vi "Lab Panel V4.86.vi"() -> ()   [LabVIEW 2013] (continued)
                    n2581 = Unbundle(w4670) -> ("DESCRIPTION"=w4650:string)  [unwired: 4 out]
                    n2582 = Unbundle(w4669) -> ("DESCRIPTION"=w4649:string)  [unwired: 4 out]
                    n2583 = Unbundle(w4668) -> ("DESCRIPTION"=w4648:string)  [unwired: 4 out]
                    n2584 = Unbundle(w4665) -> ("DESCRIPTION"=w4645:string)  [unwired: 4 out]
                    n2585 = Unbundle(w4671) -> ("DESCRIPTION"=w4651:string)  [unwired: 4 out]
                    n2586 = Unbundle(w4667) -> ("DESCRIPTION"=w4647:string)  [unwired: 4 out]
                    n2587 = Unbundle(w4674) -> ("DESCRIPTION"=w4663:string)  [unwired: 4 out]
                    n2588 = Unbundle(w4672) -> ("DESCRIPTION"=w4652:string)  [unwired: 4 out]
                    n2589 = Unbundle(w4666) -> ("DESCRIPTION"=w4646:string)  [unwired: 4 out]
                    n2590 = Unbundle(w4673) -> ("DESCRIPTION"=w4653:string)  [unwired: 4 out]
                    n2591 = Concatenate Strings("[LAB05-2/", w4645) -> (w4635:string)
                    n2592 = Concatenate Strings("[LAB05-1/", w4646) -> (w4636:string)
                    n2593 = Concatenate Strings("[LAB04-2/", w4647) -> (w4637:string)
                    n2594 = Concatenate Strings("[LAB03-2/", w4649) -> (w4639:string)
                    n2595 = Concatenate Strings("[LAB04-1/", w4648) -> (w4638:string)
                    n2596 = Concatenate Strings("[LAB03-1/", w4650) -> (w4640:string)
                    n2597 = Concatenate Strings("[LAB01-2/", w4653) -> (w4643:string)
                    n2598 = Concatenate Strings("[LAB02-2/", w4651) -> (w4641:string)
                    n2599 = Concatenate Strings("[LAB01-1/", w4663) -> (w4644:string)
                    n2600 = Concatenate Strings("[LAB02-1/", w4652) -> (w4642:string)
                  }
                  frame #1 {
                    w4698 = "/"
                    w4699 = 2.0
                    n2601 = local read "DISP LAB01-2"() -> (w4778:T4)
                    n2602 = local read "DISP LAB01-1"() -> (w4779:T4)
                    n2603 = local read "DISP LAB02-1"() -> (w4777:T4)
                    n2604 = local read "DISP LAB03-2"() -> (w4774:T4)
                    n2605 = local read "DISP LAB02-2"() -> (w4776:T4)
                    n2606 = local read "DISP LAB03-1"() -> (w4775:T4)
                    n2607 = local read "DISP LAB04-2"() -> (w4772:T4)
                    n2608 = local read "DISP LAB04-1"() -> (w4773:T4)
                    n2609 = local read "DISP LAB05-1"() -> (w4771:T4)
                    n2610 = local read "DISP LAB05-2"() -> (w4770:T4)
                    n2611 = Unbundle(w4778) -> ("CYCLE"=w4762:dbl, "MINS"=w4761:dbl, "STATUS"=w4758:string)
                    n2612 = Unbundle(w4779) -> ("CYCLE"=w4767:dbl, "MINS"=w4766:dbl, "STATUS"=w4763:string)
                    n2613 = Unbundle(w4777) -> ("CYCLE"=w4755:dbl, "MINS"=w4754:dbl, "STATUS"=w4753:string)
                    n2614 = Unbundle(w4774) -> ("CYCLE"=w4742:dbl, "MINS"=w4741:dbl, "STATUS"=w4738:string)
                    n2615 = Unbundle(w4775) -> ("CYCLE"=w4747:dbl, "MINS"=w4746:dbl, "STATUS"=w4743:string)
                    n2616 = Unbundle(w4776) -> ("CYCLE"=w4752:dbl, "MINS"=w4751:dbl, "STATUS"=w4748:string)
                    n2617 = Unbundle(w4773) -> ("CYCLE"=w4737:dbl, "MINS"=w4736:dbl, "STATUS"=w4733:string)
                    n2618 = Unbundle(w4772) -> ("CYCLE"=w4732:dbl, "MINS"=w4731:dbl, "STATUS"=w4728:string)
                    n2619 = Unbundle(w4771) -> ("CYCLE"=w4727:dbl, "MINS"=w4726:dbl, "STATUS"=w4723:string)
                    n2620 = Unbundle(w4770) -> ("CYCLE"=w4769:dbl, "MINS"=w4768:dbl, "STATUS"=w4720:string)
                    n2621 = Number To Decimal String(number=w4755) -> (decimal integer string=w4757:string)  [unwired: 1 in]
                    n2622 = Number To Decimal String(number=w4752) -> (decimal integer string=w4750:string)  [unwired: 1 in]
                    n2623 = Number To Decimal String(number=w4747) -> (decimal integer string=w4745:string)  [unwired: 1 in]
                    n2624 = Number To Decimal String(number=w4762) -> (decimal integer string=w4760:string)  [unwired: 1 in]
                    n2625 = Number To Decimal String(number=w4742) -> (decimal integer string=w4740:string)  [unwired: 1 in]
                    n2626 = Number To Decimal String(number=w4767) -> (decimal integer string=w4765:string)  [unwired: 1 in]
                    n2627 = Number To Decimal String(number=w4769) -> (decimal integer string=w4722:string)  [unwired: 1 in]
                    n2628 = Number To Decimal String(number=w4737) -> (decimal integer string=w4735:string)  [unwired: 1 in]
                    n2629 = Number To Decimal String(number=w4732) -> (decimal integer string=w4730:string)  [unwired: 1 in]
                    n2630 = Number To Decimal String(number=w4727) -> (decimal integer string=w4725:string)  [unwired: 1 in]
                    n2631 = Number To Fractional String(number=w4754, precision (6)=w4699) -> (F-format string=w4756:string)  [unwired: 2 in]
                    n2632 = Number To Fractional String(number=w4741, precision (6)=w4699) -> (F-format string=w4739:string)  [unwired: 2 in]
                    n2633 = Number To Fractional String(number=w4751, precision (6)=w4699) -> (F-format string=w4749:string)  [unwired: 2 in]
                    n2634 = Number To Fractional String(number=w4746, precision (6)=w4699) -> (F-format string=w4744:string)  [unwired: 2 in]
                    n2635 = Number To Fractional String(number=w4731, precision (6)=w4699) -> (F-format string=w4729:string)  [unwired: 2 in]
                    n2636 = Number To Fractional String(number=w4736, precision (6)=w4699) -> (F-format string=w4734:string)  [unwired: 2 in]
                    n2637 = Number To Fractional String(number=w4761, precision (6)=w4699) -> (F-format string=w4759:string)  [unwired: 2 in]
                    n2638 = Number To Fractional String(number=w4726, precision (6)=w4699) -> (F-format string=w4724:string)  [unwired: 2 in]
                    n2639 = Number To Fractional String(number=w4766, precision (6)=w4699) -> (F-format string=w4764:string)  [unwired: 2 in]
                    n2640 = Number To Fractional String(number=w4768, precision (6)=w4699) -> (F-format string=w4721:string)  [unwired: 2 in]
                    n2641 = Concatenate Strings(w4698, w4740, w4698, w4739, w4698, w4738) -> (w4714:string)
                    n2642 = Concatenate Strings(w4698, w4735, w4698, w4734, w4698, w4733) -> (w4713:string)
                    n2643 = Concatenate Strings(w4698, w4730, w4698, w4729, w4698, w4728) -> (w4712:string)
                    n2644 = Concatenate Strings(w4698, w4725, w4698, w4724, w4698, w4723) -> (w4711:string)
                    n2645 = Concatenate Strings(w4698, w4722, w4698, w4721, w4698, w4720) -> (w4710:string)
                    n2646 = Concatenate Strings(w4698, w4765, w4698, w4764, w4698, w4763) -> (w4719:string)
                    n2647 = Concatenate Strings(w4698, w4745, w4698, w4744, w4698, w4743) -> (w4715:string)
                    n2648 = Concatenate Strings(w4698, w4760, w4698, w4759, w4698, w4758) -> (w4718:string)
                    n2649 = Concatenate Strings(w4698, w4757, w4698, w4756, w4698, w4753) -> (w4717:string)
                    n2650 = Concatenate Strings(w4698, w4750, w4698, w4749, w4698, w4748) -> (w4716:string)
                    n2651 = Concatenate Strings("]", "\r") -> (w4695:string)
                    n2652 = Concatenate Strings(w4690, w4715, w4695) -> (w4705:string)
                    n2653 = Concatenate Strings(w4692, w4717, w4695) -> (w4707:string)
                    n2654 = Concatenate Strings(w4691, w4716, w4695) -> (w4706:string)
                    n2655 = Concatenate Strings(w4687, w4712, w4695) -> (w4702:string)
                    n2656 = Concatenate Strings(w4688, w4711, w4695) -> (w4703:string)
                    n2657 = Concatenate Strings(w4686, w4713, w4695) -> (w4701:string)
                    n2658 = Concatenate Strings(w4685, w4714, w4695) -> (w4700:string)
                    n2659 = Concatenate Strings(w4689, w4710, w4695) -> (w4704:string)
                    n2660 = Concatenate Strings(w4693, w4718, w4695) -> (w4708:string)
                    n2661 = Concatenate Strings(w4694, w4719, w4695) -> (w4709:string)
                    n2662 = Concatenate Strings(w4709, w4708, w4707, w4706, w4705, w4700, w4701, w4702, w4703, w4704) -> (w4678:string)
                    n2663 = Concatenate Strings("[PANEL/", "DESC/", "CYCLES/", "MINS/", "STATUS]", "\r", w4678) -> (w4677:string)
                    "MAIL REPORT" <- w4677
                    n2664 = global write "Global display 3.vi" "log all"(w4677) -> ()
                  }
                  frame #2 {
                    w4808 = "END"
                    n2665 = local read "mail control"() -> (w4809:string)
                    n2666 = case shown="False" w4804 {
                      tunnel: w4809 -> [w4833 _]
                      tunnel: w4808 -> [w4832 _]
                      tunnel: [w4831 FALSE] -> w4794
                      frame False {
                        n2667 = Equal?(x=w4833, y=w4832) -> (x = y?=w4831:bool)
                      }
                      frame True {
                      }
                    }
                    n2668 = case shown="False" w4810 {
                      tunnel: w4809 -> [w4849 _]
                      tunnel: w4808 -> [w4848 _]
                      tunnel: [w4847 FALSE] -> w4798
                      frame False {
                        n2669 = Equal?(x=w4849, y=w4848) -> (x = y?=w4847:bool)
                      }
                      frame True {
                      }
                    }
                    n2670 = case shown="False" w4807 {
                      tunnel: w4809 -> [w4845 _]
                      tunnel: w4808 -> [w4844 _]
                      tunnel: [w4843 FALSE] -> w4797
                      frame False {
                        n2671 = Equal?(x=w4845, y=w4844) -> (x = y?=w4843:bool)
                      }
                      frame True {
                      }
                    }
                    n2672 = case shown="False" w4805 {
                      tunnel: w4809 -> [w4837 _]
                      tunnel: w4808 -> [w4836 _]
                      tunnel: [w4835 FALSE] -> w4795
                      frame False {
                        n2673 = Equal?(x=w4837, y=w4836) -> (x = y?=w4835:bool)
                      }
                      frame True {
                      }
                    }
                    n2674 = case shown="False" w4806 {
                      tunnel: w4809 -> [w4841 _]
                      tunnel: w4808 -> [w4840 _]
                      tunnel: [w4839 FALSE] -> w4796
                      frame False {
                        n2675 = Equal?(x=w4841, y=w4840) -> (x = y?=w4839:bool)
                      }
                      frame True {
                      }
                    }
                    n2676 = Or(x=w4796, y=w4795) -> (x .or. y?=w4787:bool)
                    n2677 = Or(x=w4798, y=w4797) -> (x .or. y?=w4788:bool)
                    n2678 = Or(x=w4788, y=w4787) -> (x .or. y?=w4783:bool)
                    n2679 = case shown="False" w4800 {
                      tunnel: w4809 -> [w4817 _]
                      tunnel: w4808 -> [w4816 _]
                      tunnel: [w4815 FALSE] -> w4789
                      frame False {
                        n2680 = Equal?(x=w4817, y=w4816) -> (x = y?=w4815:bool)
                      }
                      frame True {
                      }
                    }
                    n2681 = case shown="False" w4799 {
                      tunnel: w4809 -> [w4813 _]
                      tunnel: w4808 -> [w4812 _]
                      tunnel: [w4811 FALSE] -> w4793
                      frame False {
                        n2682 = Equal?(x=w4813, y=w4812) -> (x = y?=w4811:bool)
                      }
                      frame True {
                      }
                    }
                    n2683 = case shown="False" w4801 {
                      tunnel: w4809 -> [w4821 _]
                      tunnel: w4808 -> [w4820 _]
                      tunnel: [w4819 FALSE] -> w4790
                      frame False {
                        n2684 = Equal?(x=w4821, y=w4820) -> (x = y?=w4819:bool)
                      }
                      frame True {
                      }
                    }
                    n2685 = case shown="False" w4803 {
                      tunnel: w4809 -> [w4829 _]
                      tunnel: w4808 -> [w4828 _]
                      tunnel: [w4827 FALSE] -> w4792
                      frame False {
                        n2686 = Equal?(x=w4829, y=w4828) -> (x = y?=w4827:bool)
                      }
                      frame True {
                      }
                    }
                    n2687 = case shown="False" w4802 {
                      tunnel: w4809 -> [w4825 _]
                      tunnel: w4808 -> [w4824 _]
                      tunnel: [w4823 FALSE] -> w4791
                      frame False {
                        n2688 = Equal?(x=w4825, y=w4824) -> (x = y?=w4823:bool)
                      }
                      frame True {
                      }
                    }
                    n2689 = Or(x=w4792, y=w4791) -> (x .or. y?=w4786:bool)
                    n2690 = Or(x=w4790, y=w4789) -> (x .or. y?=w4785:bool)
                    n2691 = Or(x=w4793, y=w4794) -> (x .or. y?=w4781:bool)
                    n2692 = Or(x=w4786, y=w4785) -> (x .or. y?=w4784:bool)
                    n2693 = Or(x=w4783, y=w4784) -> (x .or. y?=w4782:bool)
                    n2694 = Or(x=w4782, y=w4781) -> (x .or. y?=w4780:bool)
                  }
                  frame #3 {
                    n2695 = local read "on loops"() -> (w4863:dbl)
                    n2696 = local read "jig cycle"() -> (w4860:dbl)
                    n2697 = local read "Send Mail Now"() -> (w4854:bool)
                    n2698 = Add(x=w4863, y=3.0) -> (x+y=w4861:dbl)
                    n2699 = Equal?(x=w4860, y=w4861) -> (x = y?=w4855:bool)
                    n2700 = And(x=w4855, y=w4854) -> (x .and. y?=w4853:bool)
                    n2701 = And(x=w4859, y=w4855) -> (x .and. y?=w4858:bool)
                    n2702 = And(x=w4858, y=w4857) -> (x .and. y?=w4856:bool)
                    n2703 = Or(x=w4856, y=w4853) -> (x .or. y?=w4852:bool)
                    n2704 = case shown="True" w4852 {
                      tunnel: w4868 -> [_ w4874]
                      tunnel: w4867 -> [_ w4873]
                      tunnel: "Lab Panel Test Status" -> [_ w4872]
                      tunnel: w4865 -> [_ w4871]
                      tunnel: w4864 -> [_ w4870]
                      tunnel: w4851 -> [_ w4869]
                      frame False {
                      }
                      frame True {
                        n2705 = stacked-sequence {
                          tunnel: w4874 -> [w4882 _]
                          tunnel: w4873 -> [w4881 _]
                          tunnel: w4872 -> [w4880 _]
                          tunnel: w4871 -> [w4879 _]
                          tunnel: w4870 -> [w4878 _]
                          tunnel: w4869 -> [w4877 _]
                          frame #0 {
                            n2706 = call "sub vi - send mail v5.vi"("TO:"=w4882, "subject"=w4880, "from"=w4878, "out going server"=w4879, "message"=w4881) -> ("error out"=w4876:errorcluster)  [unwired: 10 in]
                            n2707 = Bundle(cluster=w4877, "mail error"=w4876) -> (w4875:T6)  [unwired: 6 in]
                            n2708 = local write "MAIL SETTINGS"(w4875) -> ()
                          }
                          frame #1 {
                            n2709 = local write "mail control"("") -> ()
                            n2710 = local write "Send Mail Now"(FALSE) -> ()
                          }
                        }
                      }
                    }
                  }
                }
              }
            }
          }
          frame #18 {
            # "save jig cycle values once all run switches are off"
            n2711 = stacked-sequence {
              tunnel: w4894 -> [_ w4923]
              tunnel: w4893 -> [_ w4922]
              tunnel: w4892 -> [_ w4921]
              tunnel: w4891 -> [_ w4920]
              tunnel: w4890 -> [_ w4919]
              tunnel: w4889 -> [_ w4918]
              tunnel: w4888 -> [_ w4917]
              tunnel: w4887 -> [_ w4916]
              tunnel: w4886 -> [_ w4915]
              tunnel: w4885 -> [_ w4914]
              frame #0 {
              }
              frame #1 {
                n2712 = Not(x=w4914) -> (.not. x?=w4897:bool)
                n2713 = Not(x=w4922) -> (.not. x?=w4912:bool)
                n2714 = Not(x=w4919) -> (.not. x?=w4907:bool)
                n2715 = Not(x=w4917) -> (.not. x?=w4903:bool)
                n2716 = Not(x=w4915) -> (.not. x?=w4899:bool)
                n2717 = Not(x=w4923) -> (.not. x?=w4913:bool)
                n2718 = Not(x=w4921) -> (.not. x?=w4911:bool)
                n2719 = Not(x=w4918) -> (.not. x?=w4905:bool)
                n2720 = Not(x=w4920) -> (.not. x?=w4909:bool)
                n2721 = Not(x=w4916) -> (.not. x?=w4901:bool)
                n2722 = local read "Save JC"() -> (w4925:bool)
                n2723 = And(x=w4913, y=w4912) -> (x .and. y?=w4910:bool)
                n2724 = And(x=w4910, y=w4911) -> (x .and. y?=w4908:bool)
                n2725 = And(x=w4908, y=w4909) -> (x .and. y?=w4906:bool)
                n2726 = And(x=w4906, y=w4907) -> (x .and. y?=w4904:bool)
                n2727 = And(x=w4904, y=w4905) -> (x .and. y?=w4902:bool)
                n2728 = And(x=w4902, y=w4903) -> (x .and. y?=w4900:bool)
                n2729 = And(x=w4900, y=w4901) -> (x .and. y?=w4898:bool)
                n2730 = And(x=w4898, y=w4899) -> (x .and. y?=w4896:bool)
                n2731 = And(x=w4896, y=w4897) -> (x .and. y?=w4895:bool)
                n2732 = And(x=w4895, y=w4925) -> (x .and. y?=w4924:bool)
                n2733 = case shown="True" w4924 {
                  tunnel: w4895 -> [w4926 _]
                  frame False {
                    n2734 = case shown="False" w4926 {
                      frame False {
                        n2735 = local write "Save JC"(TRUE) -> ()
                      }
                      frame True {
                      }
                    }
                  }
                  frame True {
                    n2736 = stacked-sequence {
                      frame #0 {
                        n2737 = String To Path(string="c:\\crabtree\\Jig Cycles\\") -> (path=w4938:path)
                        n2738 = Build Path(base path=w4938, name or relative path="jigcycles.bin") -> (appended path=w4936:path)
                        n2739 = Create Folder(path (use dialog)=w4938) -> (error out=w4940:errorcluster)  [unwired: 2 in, 2 out]
                        n2740 = local read "JIG RELAY CYCLES"() -> (w4930:T7)
                        n2741 = call <vilib>:"Clear Errors.vi"("error in (no error)"=w4940) -> ()  [unwired: 6 in, 1 out]
                        n2742 = local write "Save JC"(FALSE) -> ()
                        n2743 = Open/Create/Replace File(file path (use dialog)=w4936, operation (0:open)=T19."replace or create") -> (refnum out=w4934:refnum<file>, error out=w4935:errorcluster)  [unwired: 4 in, 1 out]
                        n2744 = Write to Binary File(file (use dialog)=w4934, data=w4930, error in=w4935) -> (refnum out=w4933:refnum<file>, error out=w4932:errorcluster)  [unwired: 3 in, 1 out]
                        n2745 = Close File(refnum=w4933, error in=w4932) -> (error out=w4931:errorcluster)  [unwired: 1 out]
                        n2746 = local write "data file error"(w4931) -> ()
                      }
                      frame #1 {
                        n2747 = local read "JIG RELAY CYCLES"() -> (w4963:T7)
                        n2748 = Unbundle By Name(w4963) -> ("LAB01-1"=w4958:dbl, "LAB01-2"=w4957:dbl, "LAB02-1"=w4955:dbl, "LAB02-2"=w4954:dbl, "LAB03-1"=w4952:dbl, "LAB03-2"=w4949:dbl, "LAB04-1"=w4948:dbl, "LAB04-2"=w4946:dbl, "LAB05-1"=w4944:dbl, "LAB05-2"=w4942:dbl)
                        n2749 = stacked-sequence {
                          tunnel: w4958 -> [w4966 _ _ _ _ _ _ _ _ _]
                          tunnel: 1000000 -> [w4969 w4979 w4989 w4999 w5009 w5019 w5029 w5039 w5049 w5059]
                          tunnel: [w4967 _ _ _ _ _ _ _ _ _] -> w4961
                          tunnel: "TEST STATION HAS REACHED 1 MILLION CYCLES, REPLACE  CONTROL RELAYS" -> [w4965 w4977 w4987 w4997 w5007 w5017 w5027 w5037 w5047 w5057]
                          tunnel: [_ w4976 _ _ _ _ _ _ _ _] -> w4959
                          tunnel: w4957 -> [_ w4975 _ _ _ _ _ _ _ _]
                          tunnel: [_ _ w4986 _ _ _ _ _ _ _] -> w4956
                          tunnel: w4955 -> [_ _ w4985 _ _ _ _ _ _ _]
                          tunnel: w4954 -> [_ _ _ w4996 _ _ _ _ _ _]
                          tunnel: [_ _ _ w4995 _ _ _ _ _ _] -> w4953
                          tunnel: w4952 -> [_ _ _ _ w5006 _ _ _ _ _]
                          tunnel: [_ _ _ _ w5005 _ _ _ _ _] -> w4951
                          tunnel: [_ _ _ _ _ w5016 _ _ _ _] -> w4950
                          tunnel: w4949 -> [_ _ _ _ _ w5015 _ _ _ _]
                          tunnel: w4948 -> [_ _ _ _ _ _ w5026 _ _ _]
                          tunnel: [_ _ _ _ _ _ w5025 _ _ _] -> w4947
                          tunnel: w4946 -> [_ _ _ _ _ _ _ w5036 _ _]
                          tunnel: [_ _ _ _ _ _ _ w5035 _ _] -> w4945
                          tunnel: w4944 -> [_ _ _ _ _ _ _ _ w5046 _]
                          tunnel: [_ _ _ _ _ _ _ _ w5045 _] -> w4943
                          tunnel: w4942 -> [_ _ _ _ _ _ _ _ _ w5056]
                          tunnel: [_ _ _ _ _ _ _ _ _ w5055] -> w4941
                          frame #0 {
                            n2750 = Greater?(x=w4966, y=w4969) -> (0:w4968:bool)
                            n2751 = case shown="True" w4968 {
                              tunnel: [w4970 0] -> w4967
                              tunnel: w4966 -> [w4970 _]
                              tunnel: w4965 -> [_ w4971]
                              frame False {
                              }
                              frame True {
                                n2752 = Concatenate Strings("LA01-1 ", w4971) -> (w4974:string)
                                n2753 = One Button Dialog(message=w4974) -> ()  [unwired: 1 in, 1 out]
                              }
                            }
                          }
                          frame #1 {
                            n2754 = Greater?(x=w4975, y=w4979) -> (0:w4978:bool)
                            n2755 = case shown="True" w4978 {
                              tunnel: [w4980 0] -> w4976
                              tunnel: w4975 -> [w4980 _]
                              tunnel: w4977 -> [_ w4981]
                              frame False {
                              }
                              frame True {
                                n2756 = Concatenate Strings("LA01-2 ", w4981) -> (w4984:string)
                                n2757 = One Button Dialog(message=w4984) -> ()  [unwired: 1 in, 1 out]
                              }
                            }
                          }
                          frame #2 {
                            n2758 = Greater?(x=w4985, y=w4989) -> (0:w4988:bool)
                            n2759 = case shown="True" w4988 {
                              tunnel: [w4990 0] -> w4986
                              tunnel: w4985 -> [w4990 _]
                              tunnel: w4987 -> [_ w4991]
                              frame False {
                              }
                              frame True {
                                n2760 = Concatenate Strings("LA02-1 ", w4991) -> (w4994:string)
                                n2761 = One Button Dialog(message=w4994) -> ()  [unwired: 1 in, 1 out]
                              }
                            }
                          }
                          frame #3 {
                            n2762 = Greater?(x=w4996, y=w4999) -> (0:w4998:bool)
                            n2763 = case shown="True" w4998 {
                              tunnel: [w5000 0] -> w4995
                              tunnel: w4996 -> [w5000 _]
                              tunnel: w4997 -> [_ w5001]
                              frame False {
                              }
                              frame True {
                                n2764 = Concatenate Strings("LA02-2 ", w5001) -> (w5004:string)
                                n2765 = One Button Dialog(message=w5004) -> ()  [unwired: 1 in, 1 out]
                              }
                            }
                          }
                          frame #4 {
                            n2766 = Greater?(x=w5006, y=w5009) -> (0:w5008:bool)
                            n2767 = case shown="True" w5008 {
                              tunnel: [w5010 0] -> w5005
                              tunnel: w5006 -> [w5010 _]
                              tunnel: w5007 -> [_ w5011]
                              frame False {
                              }
                              frame True {
                                n2768 = Concatenate Strings("LA03-1 ", w5011) -> (w5014:string)
                                n2769 = One Button Dialog(message=w5014) -> ()  [unwired: 1 in, 1 out]
                              }
                            }
                          }
                          frame #5 {
                            n2770 = Greater?(x=w5015, y=w5019) -> (0:w5018:bool)
                            n2771 = case shown="True" w5018 {
                              tunnel: [w5020 0] -> w5016
                              tunnel: w5015 -> [w5020 _]
                              tunnel: w5017 -> [_ w5021]
                              frame False {
                              }
                              frame True {
                                n2772 = Concatenate Strings("LA03-2 ", w5021) -> (w5024:string)
                                n2773 = One Button Dialog(message=w5024) -> ()  [unwired: 1 in, 1 out]
                              }
                            }
                          }
                          frame #6 {
                            n2774 = Greater?(x=w5026, y=w5029) -> (0:w5028:bool)
                            n2775 = case shown="True" w5028 {
                              tunnel: [w5030 0] -> w5025
                              tunnel: w5026 -> [w5030 _]
                              tunnel: w5027 -> [_ w5031]
                              frame False {
                              }
                              frame True {
                                n2776 = Concatenate Strings("LA04-1 ", w5031) -> (w5034:string)
                                n2777 = One Button Dialog(message=w5034) -> ()  [unwired: 1 in, 1 out]
                              }
                            }
                          }
                          frame #7 {
                            n2778 = Greater?(x=w5036, y=w5039) -> (0:w5038:bool)
                            n2779 = case shown="True" w5038 {
                              tunnel: [w5040 0] -> w5035
                              tunnel: w5036 -> [w5040 _]
                              tunnel: w5037 -> [_ w5041]
                              frame False {
                              }
                              frame True {
                                n2780 = Concatenate Strings("LA04-2 ", w5041) -> (w5044:string)
                                n2781 = One Button Dialog(message=w5044) -> ()  [unwired: 1 in, 1 out]
                              }
                            }
                          }
                          frame #8 {
                            n2782 = Greater?(x=w5046, y=w5049) -> (0:w5048:bool)
                            n2783 = case shown="True" w5048 {
                              tunnel: [w5050 0] -> w5045
                              tunnel: w5046 -> [w5050 _]
                              tunnel: w5047 -> [_ w5051]
                              frame False {
                              }
                              frame True {
                                n2784 = Concatenate Strings("LA05-1 ", w5051) -> (w5054:string)
                                n2785 = One Button Dialog(message=w5054) -> ()  [unwired: 1 in, 1 out]
                              }
                            }
                          }
                          frame #9 {
                            n2786 = Greater?(x=w5056, y=w5059) -> (0:w5058:bool)
                            n2787 = case shown="True" w5058 {
                              tunnel: [w5060 0] -> w5055
                              tunnel: w5056 -> [w5060 _]
                              tunnel: w5057 -> [_ w5061]
                              frame False {
                              }
                              frame True {
                                n2788 = Concatenate Strings("LA05-2 ", w5061) -> (w5064:string)
                                n2789 = One Button Dialog(message=w5064) -> ()  [unwired: 1 in, 1 out]
                              }
                            }
                          }
                        }
                        n2790 = Bundle By Name(cluster=w4963, "LAB01-1"=w4961, "LAB01-2"=w4959, "LAB02-1"=w4956, "LAB02-2"=w4953, "LAB03-1"=w4951, "LAB03-2"=w4950, "LAB04-1"=w4947, "LAB04-2"=w4945, "LAB05-1"=w4943, "LAB05-2"=w4941) -> (w4962:T7)
                        n2791 = local write "JIG RELAY CYCLES"(w4962) -> ()
                      }
                    }
                  }
                }
              }
            }
          }
          frame #19 {
            # "get temperature values"
            n2792 = local read "simulate"() -> (w5077:bool)
            n2793 = local read "Temp Test Cal"() -> (w5074:dbl)
            n2794 = stacked-sequence {
              tunnel: w5077 -> [_ w5133 w5178 w5223 w5268 w5313]
              tunnel: T12 {"1  (A) cal"=1.0, "1 (V) cal"=1.0, "1 (PF) cal"=1.0, "1 (TL) cal"=1.0, "1 (TN) cal"=1.0, "2 (A) cal"=1.0, "2 (V) cal"=1.0, "2 (PF) cal"=1.0, "2 (TL) cal"=1.0, "2 (TN) cal"=1.0} ("CAL LAB01") -> [_ w5132 w5177 w5222 w5267 w5312]
              tunnel: w5075 -> [_ w5130 _ _ _ _]
              tunnel: w5074 -> [_ w5126 w5176 w5221 w5266 w5311]
              tunnel: w5073 -> [_ w5121 _ _ _ _]
              tunnel: w5072 -> [_ _ w5167 _ _ _]
              tunnel: w5071 -> [_ _ w5166 _ _ _]
              tunnel: w5070 -> [_ _ _ w5212 _ _]
              tunnel: w5069 -> [_ _ _ w5211 _ _]
              tunnel: w5068 -> [_ _ _ _ w5257 _]
              tunnel: w5067 -> [_ _ _ _ w5256 _]
              tunnel: w5066 -> [_ _ _ _ _ w5302]
              tunnel: w5065 -> [_ _ _ _ _ w5301]
              frame #0 {
                n2795 = local read "Select COM port"() -> (w5082:refnum<visa-resource-name>)
                "COM port" <- w5082
                n2796 = local read "jig cycle"() -> (w5083:dbl)
                n2797 = local read "on loops"() -> (w5085:dbl)
                n2798 = global write "Global 1.vi" "tmp dly lps"("Temp Delay Lps") -> ()
                n2799 = global write "Global 1.vi" "dly value"("Temp Value") -> ()
                n2800 = Add(x=w5085, y=3) -> (x+y=w5086:dbl)
                n2801 = global write "Global 1.vi" "COM port"(w5082) -> ()
                n2802 = Equal?(x=w5083, y=w5086) -> (x = y?=w5079:bool)
                n2803 = local read "Temp Loops"() -> (w5078:dbl)
                n2804 = case shown="True" w5079 {
                  tunnel: w5078 -> [_ w5088]
                  frame False {
                  }
                  frame True {
                    n2805 = stacked-sequence {
                      tunnel: w5088 -> [w5091 w5119]
                      frame #0 {
                        n2806 = local read "simulate"() -> (w5089:bool)
                        n2807 = case shown="5" w5091 {
                          tunnel: 1.0 -> [_ w5096 w5098 w5104 w5108 w5113]
                          tunnel: w5089 -> [_ w5092 w5097 w5102 w5109 w5112]
                          frame 0, Default {
                          }
                          frame 1 {
                            w5094 = FALSE
                            n2808 = call "sub vi - GET ALL TEMP v5.vi"("LA01-EN"=TRUE, "simulate"=w5092, "LA02-EN"=w5094, "LA03-EN"=w5094, "LA04-EN"=w5094, "LA05-EN"=w5094, "Gen Cal Value"=w5096) -> ("LA01 TEMP"=w5093:T22)  [unwired: 3 in, 5 out]
                            n2809 = local write "LAB01 TEMP"(w5093) -> ()
                          }
                          frame 2 {
                            w5099 = FALSE
                            n2810 = call "sub vi - GET ALL TEMP v5.vi"("LA01-EN"=w5099, "simulate"=w5097, "LA02-EN"=TRUE, "LA03-EN"=w5099, "LA04-EN"=w5099, "LA05-EN"=w5099, "Gen Cal Value"=w5098) -> ("LA02 TEMP"=w5101:T22)  [unwired: 3 in, 5 out]
                            n2811 = local write "LAB02 TEMP"(w5101) -> ()
                          }
                          frame 3 {
                            w5105 = FALSE
                            n2812 = call "sub vi - GET ALL TEMP v5.vi"("LA01-EN"=w5105, "simulate"=w5102, "LA02-EN"=w5105, "LA03-EN"=TRUE, "LA04-EN"=w5105, "LA05-EN"=w5105, "Gen Cal Value"=w5104) -> ("LA03 TEMP"=w5103:T22)  [unwired: 3 in, 5 out]
                            n2813 = local write "LAB03 TEMP"(w5103) -> ()
                          }
                          frame 4 {
                            w5110 = FALSE
                            n2814 = call "sub vi - GET ALL TEMP v5.vi"("LA01-EN"=w5110, "simulate"=w5109, "LA02-EN"=w5110, "LA03-EN"=w5110, "LA04-EN"=TRUE, "LA05-EN"=w5110, "Gen Cal Value"=w5108) -> ("LA04 TEMP"=w5107:T22)  [unwired: 3 in, 5 out]
                            n2815 = local write "LAB04 TEMP"(w5107) -> ()
                          }
                          frame 5 {
                            w5115 = FALSE
                            n2816 = call "sub vi - GET ALL TEMP v5.vi"("LA01-EN"=w5115, "simulate"=w5112, "LA02-EN"=w5115, "LA03-EN"=w5115, "LA04-EN"=w5115, "LA05-EN"=TRUE, "Gen Cal Value"=w5113) -> ("LA05 TEMP"=w5114:T22)  [unwired: 3 in, 5 out]
                            n2817 = local write "LAB05 TEMP"(w5114) -> ()
                          }
                        }
                      }
                      frame #1 {
                        n2818 = Greater Or Equal?(x=w5119, y=5) -> (x >= y?=w5117:bool)
                        n2819 = case shown="True" w5117 {
                          frame False {
                          }
                          frame True {
                            n2820 = local write "Temp Loops"(0) -> ()
                          }
                        }
                      }
                    }
                    n2821 = local write "TEMP"(TRUE) -> ()
                  }
                }
              }
              frame #1 {
                n2822 = case shown="False" w5133 {
                  tunnel: [w5164 w5165] -> w5149
                  tunnel: w5132 -> [_ w5165]
                  frame False {
                    n2823 = local read "CAL LAB01"() -> (w5164:T12)
                  }
                  frame True {
                  }
                }
                n2824 = local read "LAB01 TEMP"() -> (w5139:T11)
                n2825 = local read "TEMP LA01"() -> (w5140:T8)
                n2826 = call "sub vi - temperature delay v2.vi"("temp values IN"=w5140, "temp signals"=w5139) -> ("T2-N"=w5135:dbl, "T2-L"=w5136:dbl, "T1-N"=w5137:dbl, "T1-L"=w5138:dbl, "temp values OUT"=w5134:T40)  [unwired: 5 in]
                n2827 = Unbundle By Name(w5149) -> ("1 (TL) cal"=w5144:dbl, "1 (TN) cal"=w5143:dbl, "2 (TL) cal"=w5142:dbl, "2 (TN) cal"=w5141:dbl)  [unwired: 6 out]
                n2828 = local write "TEMP LA01"(w5134) -> ()
                n2829 = Multiply(x=w5138, y=w5144) -> (x*y=w5131:dbl)
                n2830 = Multiply(x=w5137, y=w5143) -> (x*y=w5128:dbl)
                n2831 = Multiply(x=w5136, y=w5142) -> (x*y=w5125:dbl)
                n2832 = Multiply(x=w5135, y=w5141) -> (x*y=w5124:dbl)
                n2833 = case shown="True" w5130 {
                  tunnel: w5131 -> [w5158 w5163]
                  tunnel: w5126 -> [_ w5161]
                  tunnel: [w5158 w5162] -> w5129
                  tunnel: w5128 -> [w5157 w5160]
                  tunnel: [w5157 w5159] -> w5127
                  frame False {
                  }
                  frame True {
                    n2834 = Multiply(x=w5161, y=w5160) -> (x*y=w5159:dbl)
                    n2835 = Multiply(x=w5161, y=w5163) -> (x*y=w5162:dbl)
                  }
                }
                n2836 = case shown="True" w5121 {
                  tunnel: w5125 -> [w5151 w5156]
                  tunnel: w5126 -> [_ w5154]
                  tunnel: [w5151 w5155] -> w5123
                  tunnel: w5124 -> [w5150 w5153]
                  tunnel: [w5150 w5152] -> w5122
                  frame False {
                  }
                  frame True {
                    n2837 = Multiply(x=w5154, y=w5153) -> (x*y=w5152:dbl)
                    n2838 = Multiply(x=w5154, y=w5156) -> (x*y=w5155:dbl)
                  }
                }
                n2839 = local read "SIG LAB01-2"() -> (w5146:T2)
                n2840 = local read "SIG LAB01-1"() -> (w5148:T2)
                n2841 = Bundle By Name(cluster=w5148, "Tmp Live"=w5129, "Tmp Neut"=w5127) -> (w5147:T2)
                n2842 = Bundle By Name(cluster=w5146, "Tmp Live"=w5123, "Tmp Neut"=w5122) -> (w5145:T2)
                n2843 = local write "SIG LAB01-1"(w5147) -> ()
                n2844 = local write "SIG LAB01-2"(w5145) -> ()
              }
              frame #2 {
                n2845 = case shown="True" w5178 {
                  tunnel: [w5209 w5210] -> w5194
                  tunnel: w5177 -> [_ w5210]
                  frame False {
                    n2846 = local read "CAL LAB02"() -> (w5209:T13)
                  }
                  frame True {
                  }
                }
                n2847 = local read "LAB02 TEMP"() -> (w5185:T11)
                n2848 = local read "TEMP LA02"() -> (w5184:T8)
                n2849 = call "sub vi - temperature delay v2.vi"("temp values IN"=w5184, "temp signals"=w5185) -> ("T2-N"=w5179:dbl, "T2-L"=w5180:dbl, "T1-N"=w5181:dbl, "T1-L"=w5182:dbl, "temp values OUT"=w5183:T40)  [unwired: 5 in]
                n2850 = Unbundle By Name(w5194) -> ("1 (TL) cal"=w5189:dbl, "1 (TN) cal"=w5188:dbl, "2 (TL) cal"=w5187:dbl, "2 (TN) cal"=w5186:dbl)  [unwired: 6 out]
                n2851 = local write "TEMP LA02"(w5183) -> ()
                n2852 = Multiply(x=w5182, y=w5189) -> (x*y=w5175:dbl)
                n2853 = Multiply(x=w5181, y=w5188) -> (x*y=w5174:dbl)
                n2854 = Multiply(x=w5180, y=w5187) -> (x*y=w5171:dbl)
                n2855 = Multiply(x=w5179, y=w5186) -> (x*y=w5170:dbl)
                n2856 = case shown="True" w5167 {
                  tunnel: w5175 -> [w5203 w5208]
                  tunnel: w5176 -> [_ w5206]
                  tunnel: [w5203 w5207] -> w5173
                  tunnel: w5174 -> [w5202 w5205]
                  tunnel: [w5202 w5204] -> w5172
                  frame False {
                  }
                  frame True {
                    n2857 = Multiply(x=w5206, y=w5205) -> (x*y=w5204:dbl)
                    n2858 = Multiply(x=w5206, y=w5208) -> (x*y=w5207:dbl)
                  }
                }
                n2859 = case shown="True" w5166 {
                  tunnel: w5171 -> [w5196 w5201]
                  tunnel: w5176 -> [_ w5199]
                  tunnel: [w5196 w5200] -> w5169
                  tunnel: w5170 -> [w5195 w5198]
                  tunnel: [w5195 w5197] -> w5168
                  frame False {
                  }
                  frame True {
                    n2860 = Multiply(x=w5199, y=w5198) -> (x*y=w5197:dbl)
                    n2861 = Multiply(x=w5199, y=w5201) -> (x*y=w5200:dbl)
                  }
                }
                n2862 = local read "SIG LAB02-2"() -> (w5191:T2)
                n2863 = local read "SIG LAB02-1"() -> (w5193:T2)
                n2864 = Bundle By Name(cluster=w5193, "Tmp Live"=w5173, "Tmp Neut"=w5172) -> (w5192:T2)
                n2865 = Bundle By Name(cluster=w5191, "Tmp Live"=w5169, "Tmp Neut"=w5168) -> (w5190:T2)
                n2866 = local write "SIG LAB02-1"(w5192) -> ()
                n2867 = local write "SIG LAB02-2"(w5190) -> ()
              }
              frame #3 {
                n2868 = case shown="False" w5223 {
                  tunnel: [w5254 w5255] -> w5239
                  tunnel: w5222 -> [_ w5255]
                  frame False {
                    n2869 = local read "CAL LAB03"() -> (w5254:T12)
                  }
                  frame True {
                  }
                }
                n2870 = local read "TEMP LA03"() -> (w5229:T8)
                n2871 = local read "LAB03 TEMP"() -> (w5230:T11)
                n2872 = call "sub vi - temperature delay v2.vi"("temp values IN"=w5229, "temp signals"=w5230) -> ("T2-N"=w5224:dbl, "T2-L"=w5225:dbl, "T1-N"=w5226:dbl, "T1-L"=w5227:dbl, "temp values OUT"=w5228:T40)  [unwired: 5 in]
                n2873 = Unbundle By Name(w5239) -> ("1 (TL) cal"=w5234:dbl, "1 (TN) cal"=w5233:dbl, "2 (TL) cal"=w5232:dbl, "2 (TN) cal"=w5231:dbl)  [unwired: 6 out]
                n2874 = local write "TEMP LA03"(w5228) -> ()
                n2875 = Multiply(x=w5227, y=w5234) -> (x*y=w5220:dbl)
                n2876 = Multiply(x=w5226, y=w5233) -> (x*y=w5219:dbl)
                n2877 = Multiply(x=w5225, y=w5232) -> (x*y=w5216:dbl)
                n2878 = Multiply(x=w5224, y=w5231) -> (x*y=w5215:dbl)
                n2879 = case shown="True" w5211 {
                  tunnel: w5216 -> [w5241 w5246]
                  tunnel: w5221 -> [_ w5244]
                  tunnel: [w5241 w5245] -> w5214
                  tunnel: w5215 -> [w5240 w5243]
                  tunnel: [w5240 w5242] -> w5213
                  frame False {
                  }
                  frame True {
                    n2880 = Multiply(x=w5244, y=w5243) -> (x*y=w5242:dbl)
                    n2881 = Multiply(x=w5244, y=w5246) -> (x*y=w5245:dbl)
                  }
                }
                n2882 = case shown="True" w5212 {
                  tunnel: w5220 -> [w5248 w5253]
                  tunnel: w5221 -> [_ w5251]
                  tunnel: [w5248 w5252] -> w5218
                  tunnel: w5219 -> [w5247 w5250]
                  tunnel: [w5247 w5249] -> w5217
                  frame False {
                  }
                  frame True {
                    n2883 = Multiply(x=w5251, y=w5250) -> (x*y=w5249:dbl)
                    n2884 = Multiply(x=w5251, y=w5253) -> (x*y=w5252:dbl)
                  }
                }
                n2885 = local read "SIG LAB03-2"() -> (w5236:T2)
                n2886 = local read "SIG LAB03-1"() -> (w5238:T2)
                n2887 = Bundle By Name(cluster=w5238, "Tmp Live"=w5218, "Tmp Neut"=w5217) -> (w5237:T2)
                n2888 = Bundle By Name(cluster=w5236, "Tmp Live"=w5214, "Tmp Neut"=w5213) -> (w5235:T2)
                n2889 = local write "SIG LAB03-1"(w5237) -> ()
                n2890 = local write "SIG LAB03-2"(w5235) -> ()
              }
              frame #4 {
                n2891 = case shown="False" w5268 {
                  tunnel: [w5299 w5300] -> w5284
                  tunnel: w5267 -> [_ w5300]
                  frame False {
                    n2892 = local read "CAL LAB04"() -> (w5299:T12)
                  }
                  frame True {
                  }
                }
                n2893 = local read "LAB04 TEMP"() -> (w5274:T11)
                n2894 = local read "TEMP LA04"() -> (w5275:T8)
                n2895 = call "sub vi - temperature delay v2.vi"("temp values IN"=w5275, "temp signals"=w5274) -> ("T2-N"=w5269:dbl, "T2-L"=w5270:dbl, "T1-N"=w5271:dbl, "T1-L"=w5272:dbl, "temp values OUT"=w5273:T40)  [unwired: 5 in]
                n2896 = Unbundle By Name(w5284) -> ("1 (TL) cal"=w5279:dbl, "1 (TN) cal"=w5278:dbl, "2 (TL) cal"=w5277:dbl, "2 (TN) cal"=w5276:dbl)  [unwired: 6 out]
                n2897 = local write "TEMP LA04"(w5273) -> ()
                n2898 = Multiply(x=w5272, y=w5279) -> (x*y=w5265:dbl)
                n2899 = Multiply(x=w5271, y=w5278) -> (x*y=w5264:dbl)
                n2900 = Multiply(x=w5270, y=w5277) -> (x*y=w5261:dbl)
                n2901 = Multiply(x=w5269, y=w5276) -> (x*y=w5260:dbl)
                n2902 = case shown="True" w5256 {
                  tunnel: w5261 -> [w5286 w5291]
                  tunnel: w5266 -> [_ w5289]
                  tunnel: [w5286 w5290] -> w5259
                  tunnel: w5260 -> [w5285 w5288]
                  tunnel: [w5285 w5287] -> w5258
                  frame False {
                  }
                  frame True {
                    n2903 = Multiply(x=w5289, y=w5288) -> (x*y=w5287:dbl)
                    n2904 = Multiply(x=w5289, y=w5291) -> (x*y=w5290:dbl)
                  }
                }
                n2905 = case shown="True" w5257 {
                  tunnel: w5265 -> [w5293 w5298]
                  tunnel: w5266 -> [_ w5296]
                  tunnel: [w5293 w5297] -> w5263
                  tunnel: w5264 -> [w5292 w5295]
                  tunnel: [w5292 w5294] -> w5262
                  frame False {
                  }
                  frame True {
                    n2906 = Multiply(x=w5296, y=w5295) -> (x*y=w5294:dbl)
                    n2907 = Multiply(x=w5296, y=w5298) -> (x*y=w5297:dbl)
                  }
                }
                n2908 = local read "SIG LAB04-2"() -> (w5281:T2)
                n2909 = local read "SIG LAB04-1"() -> (w5283:T2)
                n2910 = Bundle By Name(cluster=w5283, "Tmp Live"=w5263, "Tmp Neut"=w5262) -> (w5282:T2)
                n2911 = Bundle By Name(cluster=w5281, "Tmp Live"=w5259, "Tmp Neut"=w5258) -> (w5280:T2)
                n2912 = local write "SIG LAB04-1"(w5282) -> ()
                n2913 = local write "SIG LAB04-2"(w5280) -> ()
              }
              frame #5 {
                n2914 = case shown="False" w5313 {
                  tunnel: [w5344 w5345] -> w5329
                  tunnel: w5312 -> [_ w5345]
                  frame False {
                    n2915 = local read "CAL LAB05"() -> (w5344:T12)
                  }
                  frame True {
                  }
                }
                n2916 = local read "LAB05 TEMP"() -> (w5319:T11)
                n2917 = local read "TEMP LA05"() -> (w5320:T8)
                n2918 = call "sub vi - temperature delay v2.vi"("temp values IN"=w5320, "temp signals"=w5319) -> ("T2-N"=w5315:dbl, "T2-L"=w5316:dbl, "T1-N"=w5317:dbl, "T1-L"=w5318:dbl, "temp values OUT"=w5314:T40)  [unwired: 5 in]
                n2919 = local write "TEMP LA05"(w5314) -> ()
                n2920 = Unbundle By Name(w5329) -> ("1 (TL) cal"=w5321:dbl, "1 (TN) cal"=w5324:dbl, "2 (TL) cal"=w5323:dbl, "2 (TN) cal"=w5322:dbl)  [unwired: 6 out]
                n2921 = Multiply(x=w5318, y=w5321) -> (x*y=w5310:dbl)
                n2922 = Multiply(x=w5317, y=w5324) -> (x*y=w5309:dbl)
                n2923 = Multiply(x=w5316, y=w5323) -> (x*y=w5306:dbl)
                n2924 = Multiply(x=w5315, y=w5322) -> (x*y=w5305:dbl)
                n2925 = case shown="True" w5301 {
                  tunnel: w5306 -> [w5331 w5336]
                  tunnel: w5311 -> [_ w5334]
                  tunnel: [w5331 w5335] -> w5304
                  tunnel: w5305 -> [w5330 w5333]
                  tunnel: [w5330 w5332] -> w5303
                  frame False {
                  }
                  frame True {
                    n2926 = Multiply(x=w5334, y=w5333) -> (x*y=w5332:dbl)
                    n2927 = Multiply(x=w5334, y=w5336) -> (x*y=w5335:dbl)
                  }
                }
                n2928 = case shown="True" w5302 {
                  tunnel: w5310 -> [w5338 w5343]
                  tunnel: w5311 -> [_ w5341]
                  tunnel: [w5338 w5342] -> w5308
